vi "GV PreframeclockScanGalvo.vi"() -> ()   [LabVIEW 2017]
panel:
  out "PreframeclockScanGalvo":bool
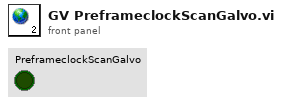
[diagram p1: front panel]
diagram:
